vi "EXA get screen shot_main.vi"() -> ()   [LabVIEW 2016]
panel:
  in  "VISA in":refnum<visa-resource-name>
  in  "File name":string
  in  "Path":path
  in  "stop":bool
  in  "Catch Screenshot":bool
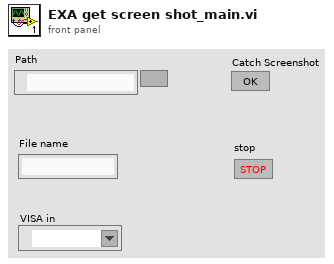
[diagram p1: front panel]
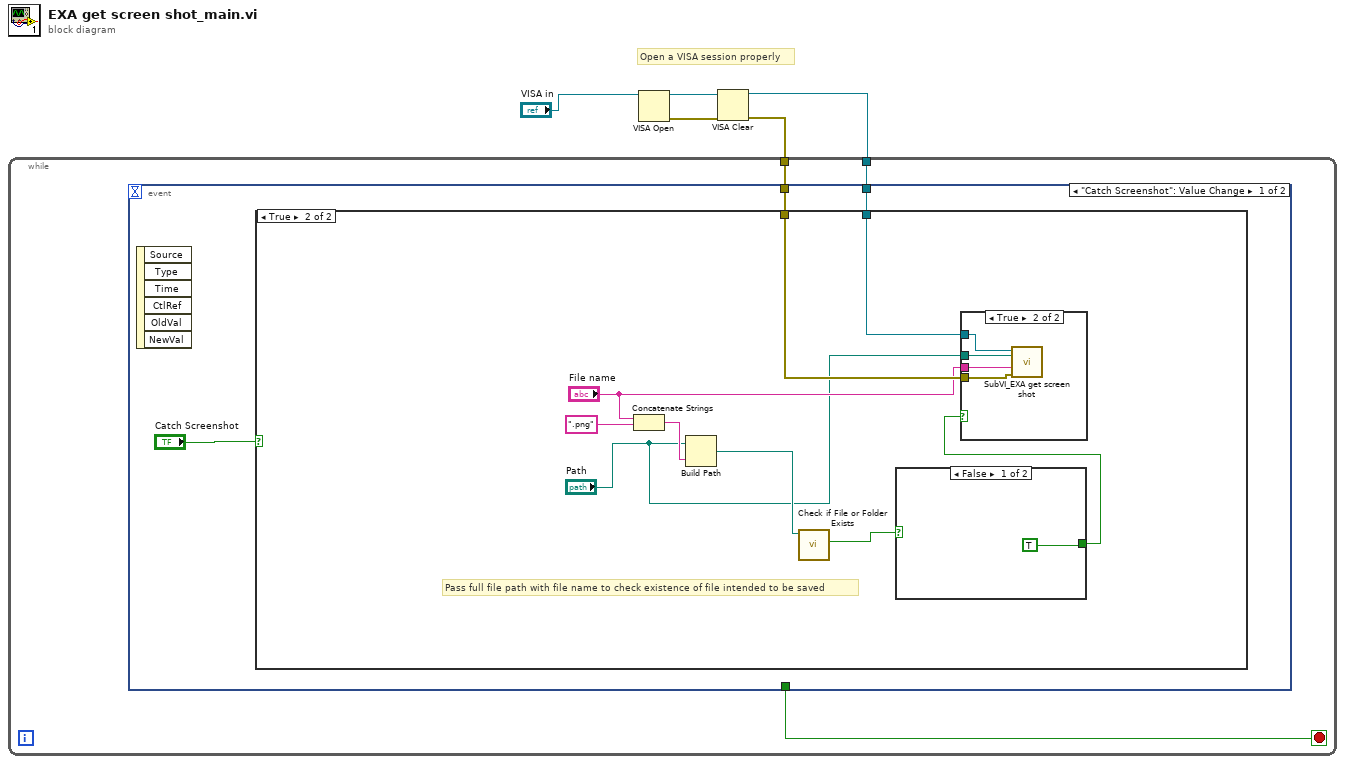
[diagram p0: block diagram]
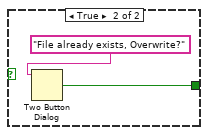
[diagram p4: hidden frame]
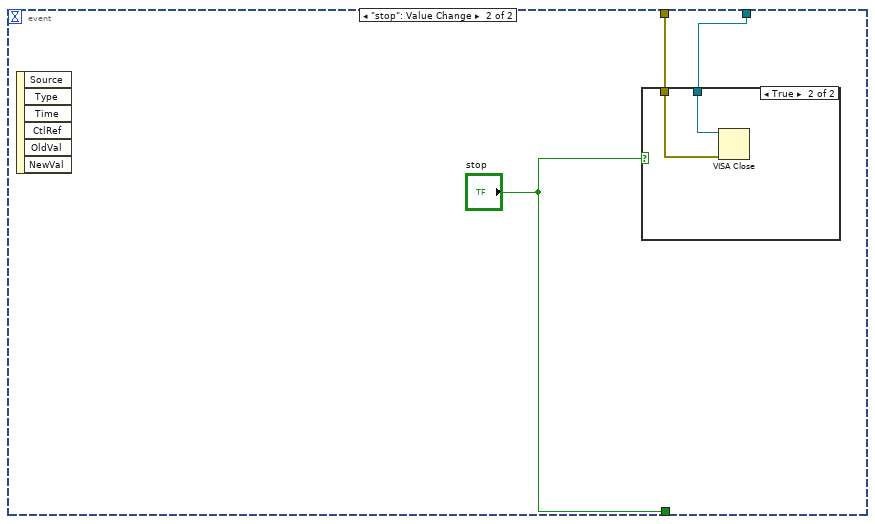
[diagram p5: hidden frame]
diagram:
  # "Open a VISA session properly"
  n1 = VISA Open(VISA resource name="VISA in") -> (VISA resource name=w4:refnum<visa-resource-name>, error out=w1:errorcluster)  [unwired: 4 in]
  n2 = VISA Clear(VISA resource name=w4, error in (no error)=w1) -> (VISA resource name out=w3:refnum<visa-resource-name>, error out=w2:errorcluster)
  n3 = while {
    tunnel: w3 -> [w7]
    tunnel: w2 -> [w6]
    stop <- w8 stop-if-true
    n4 = event shown="[0] \"Catch Screenshot\": Value Change" {
      selector: _ -> [_ _]
      dyn-events: _ -> [_ _]
      timeout: _ -> [_ _]
      tunnel: [_ "stop"] -> w8
      tunnel: w7 -> [w10 w30]
      tunnel: w6 -> [w9 w29]
      event "Catch Screenshot": Value Change {
        n5 = event-data() -> ()  [unwired: 1 in, 6 out]
        n6 = case shown="True" "Catch Screenshot" {
          tunnel: w10 -> [_ w20]
          tunnel: w9 -> [_ w19]
          frame False {
          }
          frame True {
            # "Pass full file path with file name to check existence of file intended to be saved"
            n7 = Concatenate Strings("File name", ".png") -> (w14:string)
            n8 = Build Path(base path="Path", name or relative path=w14) -> (appended path=w13:path)
            n9 = call <vilib>:"Check if File or Folder Exists.vi"("path"=w13) -> ("file or folder exists?"=w18:bool)  [unwired: 8 in, 2 out]
            n10 = case shown="False" w18 {
              tunnel: [TRUE w26] -> w17
              frame False {
              }
              frame True {
                n11 = Two Button Dialog(message="File already exists, Overwrite?") -> (T button?=w26:bool)  [unwired: 2 in]
              }
            }
            n12 = case shown="True" w17 {
              tunnel: "Path" -> [_ w24]
              tunnel: "File name" -> [_ w23]
              tunnel: w20 -> [_ w22]
              tunnel: w19 -> [_ w21]
              frame False {
              }
              frame True {
                n13 = call "SubVI_EXA get screen shot.vi"("error in (no error)"=w21, "File name"=w23, "Path"=w24, "VISA resource in"=w22) -> ()  [unwired: 6 in, 2 out]
              }
            }
          }
        }
      }
      event "stop": Value Change {
        n14 = event-data() -> ()  [unwired: 1 in, 6 out]
        n15 = case shown="True" "stop" {
          tunnel: w30 -> [_ w32]
          tunnel: w29 -> [_ w31]
          frame False {
          }
          frame True {
            n16 = VISA Close(VISA resource name=w32, error in (no error)=w31) -> ()  [unwired: 1 out]
          }
        }
      }
    }
  }
